vi "Temp_formula.vi"(3 "NTCin":dbl) -> (11 "TempOut":dbl)   [LabVIEW 2023]
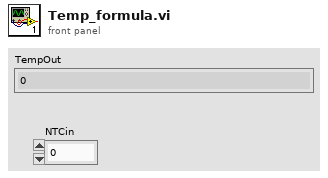
[diagram p1: front panel]
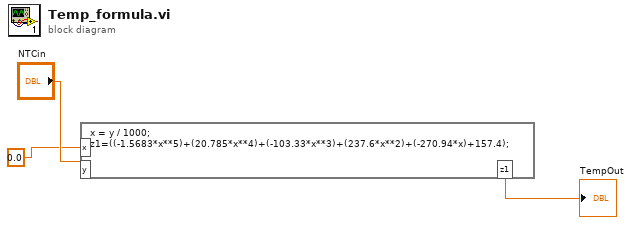
[diagram p0: block diagram]
diagram:
  n1 = formula code="x = y / 1000;\nz1=((-1.5683*x**5)+(20.785*x**4)+(-103.33*x**3)+(237.6*x**2)+(-270.94*x)+157.4);"("y"="NTCin", "x"=0.0) -> ("z1"=→"TempOut":dbl)
